vi "Prompt Password.vi"(8 "error in (no error)":errorcluster, 10 "Prompt":string="Password" caption="Prompt (\"Password\")") -> (0 "error out":errorcluster, 1 "Value":string)   [LabVIEW 2018, in "MGI-Console.lvlib" / "Console.lvclass"]
doc: "Prompts the user for input.\n\n<b>Default Value</b> is returned if the user does not enter any input (meaning they just press the enter key).\n----\nCopyright: MGI 2018\nAuthor: Derek Trepanier"
uses:
  Console.lvclass
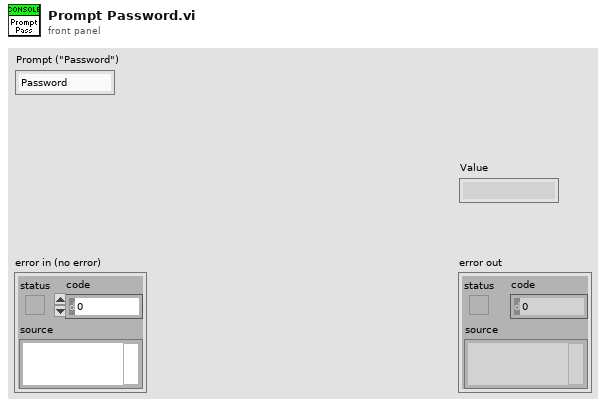
[diagram p1: front panel]
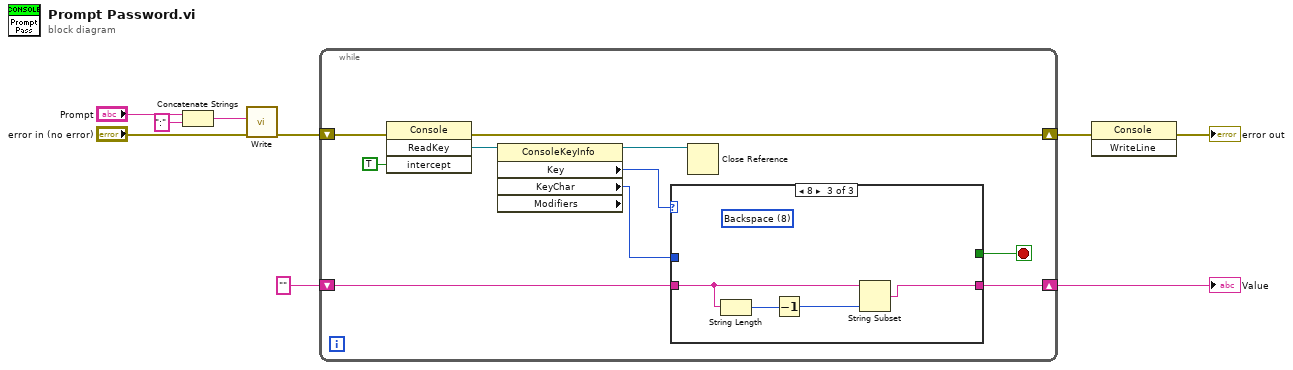
[diagram p0: block diagram]
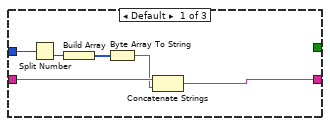
[diagram p2: hidden frame]
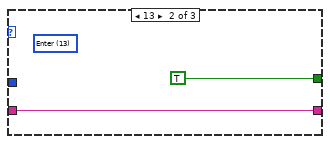
[diagram p3: hidden frame]
diagram:
  n1 = Concatenate Strings("Prompt", ":" ("string")) -> (w9:string)
  n2 = call "Write.vi"("error in (no error)"="error in (no error)", "String"=w9) -> ("error out"=w5:errorcluster)  [unwired: 9 in]
  n3 = while {
    shift-right: [w18] -> w2
    shift-left: w5 -> [w19]
    shift-right: [w11] -> w3
    shift-left: "" -> [w12]
    stop <- w13 stop-if-true
    n4 = invoke class="Console" method="ReadKey"(error in=w19, "intercept"=TRUE) -> (error out=w18:errorcluster, "ReadKey"=w17:refnum<k24>)  [unwired: 2 in, 2 out]
    n5 = property class="ConsoleKeyInfo" props=["Key", "KeyChar", "Modifiers"](reference=w17) -> (reference out=w14:refnum<k24>, "Key"=w15:i32, "KeyChar"=w10:u16)  [unwired: 1 in, 2 out]
    n6 = case shown="8" w15 {
      tunnel: [_ TRUE _] -> w13
      tunnel: w12 -> [w25 w26 w30]
      tunnel: [w24 w26 w31] -> w11
      tunnel: w10 -> [w23 _ _]
      frame Default {
        n7 = Split Number(x=w23) -> (lo(x)=w22:u8)  [unwired: 1 out]
        n8 = Build Array(w22) -> (w20:u8[])
        n9 = Byte Array To String(unsigned byte array=w20) -> (string=w21:string)
        n10 = Concatenate Strings(w25, w21) -> (w24:string)
      }
      frame 13 {
        (unwired) 13 items=["Backspace"=8, "Tab"=9, "Clear"=12, "Enter"=13, "Pause"=19, "Escape"=27, "Spacebar"=32, "PageUp"=33, "PageDown"=34, "End"=35, "Home"=36, "LeftArrow"=37, "UpArrow"=38, "RightArrow"=39, "DownArrow"=40, "Select"=41, "Print"=42, "Execute"=43, "PrintScreen"=44, "Insert"=45, "Delete"=46, "Help"=47, "D0"=48, "D1"=49, "D2"=50, "D3"=51, "D4"=52, "D5"=53, "D6"=54, "D7"=55, "D8"=56, "D9"=57, "A"=65, "B"=66, "C"=67, "D"=68, "E"=69, "F"=70, "G"=71, "H"=72, "I"=73, "J"=74, "K"=75, "L"=76, "M"=77, "N"=78, "O"=79, "P"=80, "Q"=81, "R"=82, "S"=83, "T"=84, "U"=85, "V"=86, "W"=87, "X"=88, "Y"=89, "Z"=90, "LeftWindows"=91, "RightWindows"=92, "Applications"=93, "Sleep"=95, "NumPad0"=96, "NumPad1"=97, "NumPad2"=98, "NumPad3"=99, "NumPad4"=100, "NumPad5"=101, "NumPad6"=102, "NumPad7"=103, "NumPad8"=104, "NumPad9"=105, "Multiply"=106, "Add"=107, "Separator"=108, "Subtract"=109, "Decimal"=110, "Divide"=111, "F1"=112, "F2"=113, "F3"=114, "F4"=115, "F5"=116, "F6"=117, "F7"=118, "F8"=119, "F9"=120, "F10"=121, "F11"=122, "F12"=123, "F13"=124, "F14"=125, "F15"=126, "F16"=127, "F17"=128, "F18"=129, "F19"=130, "F20"=131, "F21"=132, "F22"=133, "F23"=134, "F24"=135, "BrowserBack"=166, "BrowserForward"=167, "BrowserRefresh"=168, "BrowserStop"=169, "BrowserSearch"=170, "BrowserFavorites"=171, "BrowserHome"=172, "VolumeMute"=173, "VolumeDown"=174, "VolumeUp"=175, "MediaNext"=176, "MediaPrevious"=177, "MediaStop"=178, "MediaPlay"=179, "LaunchMail"=180, "LaunchMediaSelect"=181, "LaunchApp1"=182, "LaunchApp2"=183, "Oem1"=186, "OemPlus"=187, "OemComma"=188, "OemMinus"=189, "OemPeriod"=190, "Oem2"=191, "Oem3"=192, "Oem4"=219, "Oem5"=220, "Oem6"=221, "Oem7"=222, "Oem8"=223, "Oem102"=226, "Process"=229, "Packet"=231, "Attention"=246, "CrSel"=247, "ExSel"=248, "EraseEndOfFile"=249, "Play"=250, "Zoom"=251, "NoName"=252, "Pa1"=253, "OemClear"=254] ("Key")
      }
      frame 8 {
        (unwired) 8 items=["Backspace"=8, "Tab"=9, "Clear"=12, "Enter"=13, "Pause"=19, "Escape"=27, "Spacebar"=32, "PageUp"=33, "PageDown"=34, "End"=35, "Home"=36, "LeftArrow"=37, "UpArrow"=38, "RightArrow"=39, "DownArrow"=40, "Select"=41, "Print"=42, "Execute"=43, "PrintScreen"=44, "Insert"=45, "Delete"=46, "Help"=47, "D0"=48, "D1"=49, "D2"=50, "D3"=51, "D4"=52, "D5"=53, "D6"=54, "D7"=55, "D8"=56, "D9"=57, "A"=65, "B"=66, "C"=67, "D"=68, "E"=69, "F"=70, "G"=71, "H"=72, "I"=73, "J"=74, "K"=75, "L"=76, "M"=77, "N"=78, "O"=79, "P"=80, "Q"=81, "R"=82, "S"=83, "T"=84, "U"=85, "V"=86, "W"=87, "X"=88, "Y"=89, "Z"=90, "LeftWindows"=91, "RightWindows"=92, "Applications"=93, "Sleep"=95, "NumPad0"=96, "NumPad1"=97, "NumPad2"=98, "NumPad3"=99, "NumPad4"=100, "NumPad5"=101, "NumPad6"=102, "NumPad7"=103, "NumPad8"=104, "NumPad9"=105, "Multiply"=106, "Add"=107, "Separator"=108, "Subtract"=109, "Decimal"=110, "Divide"=111, "F1"=112, "F2"=113, "F3"=114, "F4"=115, "F5"=116, "F6"=117, "F7"=118, "F8"=119, "F9"=120, "F10"=121, "F11"=122, "F12"=123, "F13"=124, "F14"=125, "F15"=126, "F16"=127, "F17"=128, "F18"=129, "F19"=130, "F20"=131, "F21"=132, "F22"=133, "F23"=134, "F24"=135, "BrowserBack"=166, "BrowserForward"=167, "BrowserRefresh"=168, "BrowserStop"=169, "BrowserSearch"=170, "BrowserFavorites"=171, "BrowserHome"=172, "VolumeMute"=173, "VolumeDown"=174, "VolumeUp"=175, "MediaNext"=176, "MediaPrevious"=177, "MediaStop"=178, "MediaPlay"=179, "LaunchMail"=180, "LaunchMediaSelect"=181, "LaunchApp1"=182, "LaunchApp2"=183, "Oem1"=186, "OemPlus"=187, "OemComma"=188, "OemMinus"=189, "OemPeriod"=190, "Oem2"=191, "Oem3"=192, "Oem4"=219, "Oem5"=220, "Oem6"=221, "Oem7"=222, "Oem8"=223, "Oem102"=226, "Process"=229, "Packet"=231, "Attention"=246, "CrSel"=247, "ExSel"=248, "EraseEndOfFile"=249, "Play"=250, "Zoom"=251, "NoName"=252, "Pa1"=253, "OemClear"=254] ("Key")
        n11 = String Length(string=w30) -> (length=w29:i32)
        n12 = Decrement(x=w29) -> (x-1=w28:i32)
        n13 = String Subset(string=w30, length (rest)=w28) -> (substring=w31:string)  [unwired: 1 in]
      }
    }
    n14 = Close Reference(reference=w14) -> ()  [unwired: 1 in, 1 out]
  }
  "Value" <- w3
  n15 = invoke class="Console" method="WriteLine"(error in=w2) -> (error out=→"error out":errorcluster)  [unwired: 2 in, 2 out]
